vi "Parse INCAR.vi"(8 "error in (no error)":errorcluster, 11 "INCAR File":path=path "C:/Users/Chris B/Documents/Ab Initio/Vasp Calculations/Batch4_20130519/1_Again") -> (0 "error out":errorcluster, 1 "INCAR ID":string, 2 "INCAR Raw Commands":T2(array[cluster]), 3 "INCAR Summary":T1, 5 "Allow Relaxation?":bool)   [LabVIEW 2010]
uses:
  <vilib>/Utility/file.llb/Read From Spreadsheet File (string).vi
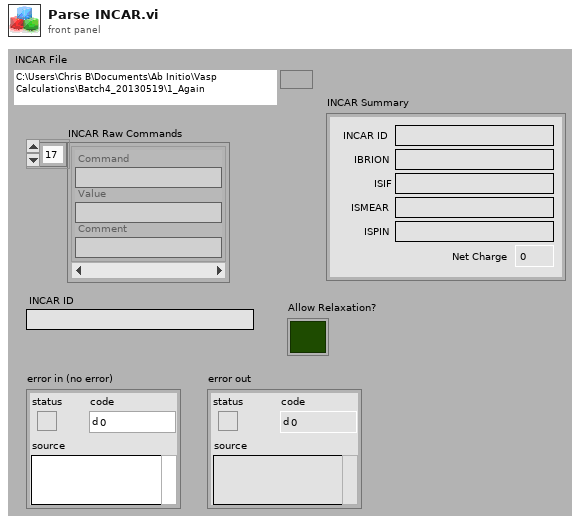
[diagram p1: front panel]
types:
  T1 = cluster{"INCAR ID":string, "IBRION":string, "ISIF":string, "ISMEAR":string, "ISPIN":string, "Net Charge":i32}
  T2 = cluster{"Command":string, "Value":string, "Comment":string}[]
  T3 = cluster{"trimmed string":string, "trimmed string":string, "trimmed string":string}
  T4 = cluster{"trimmed string":string, "trimmed string":string, "trimmed string":string}[]
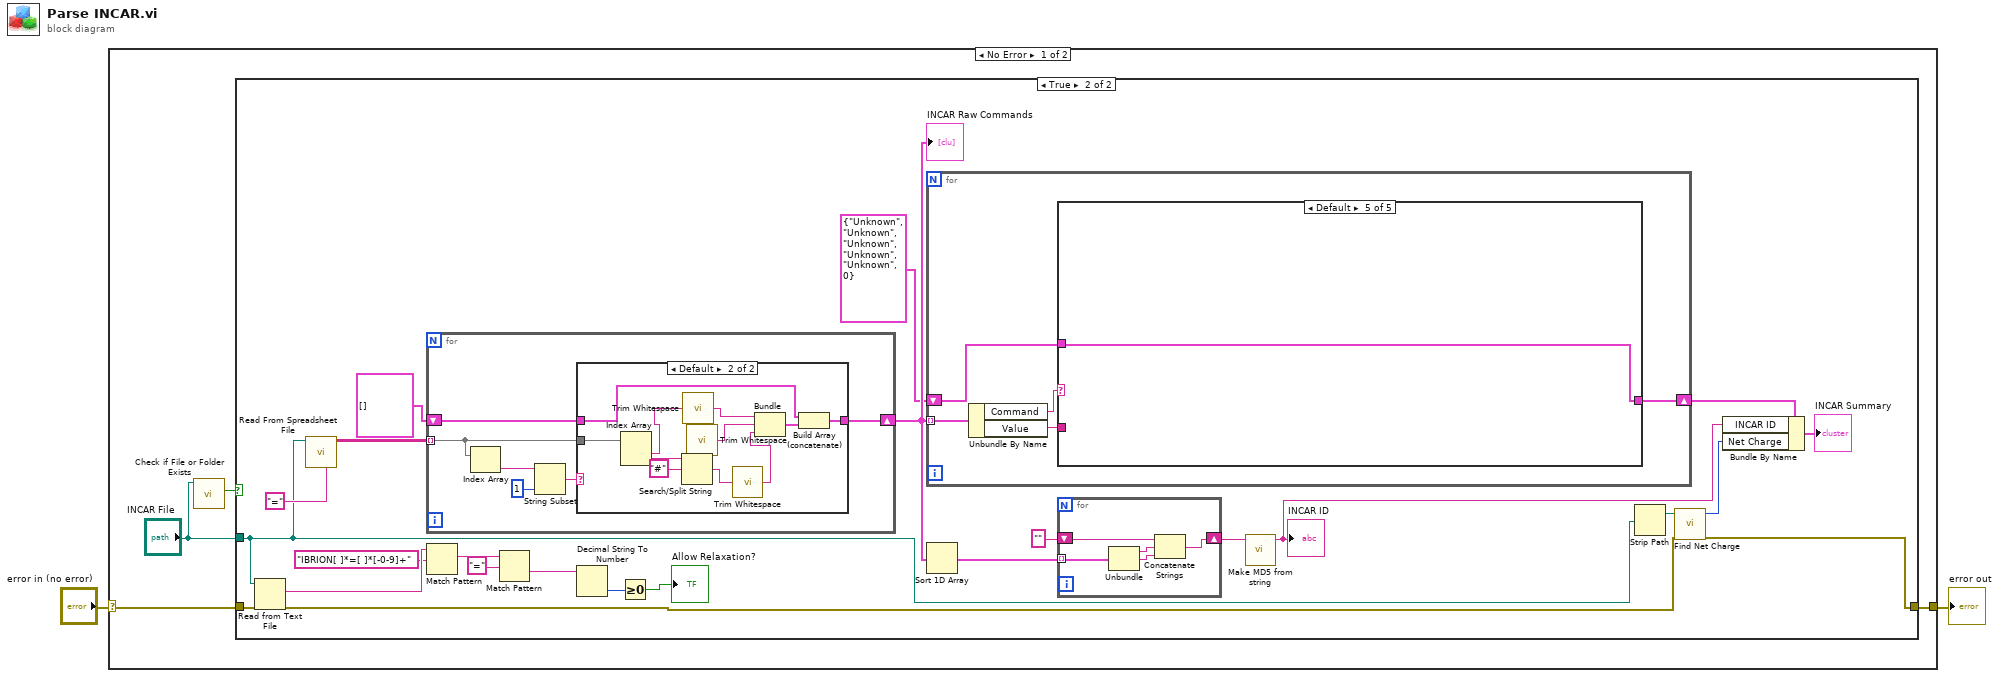
[diagram p0: block diagram]
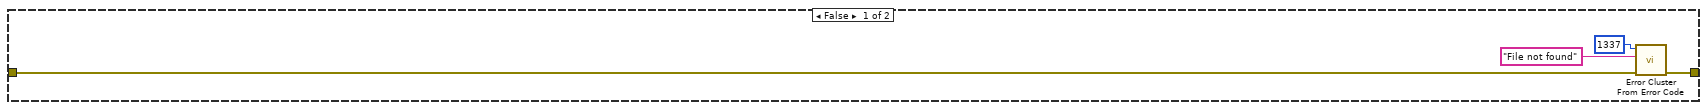
[diagram p2: hidden frame]
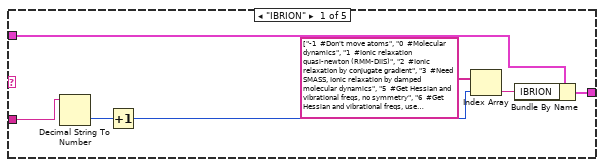
[diagram p3: hidden frame]
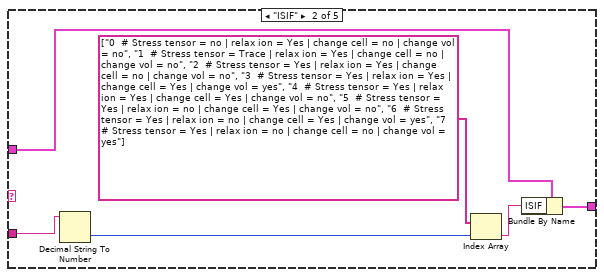
[diagram p4: hidden frame]
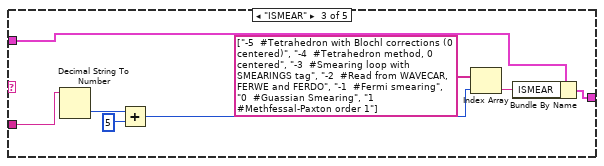
[diagram p5: hidden frame]
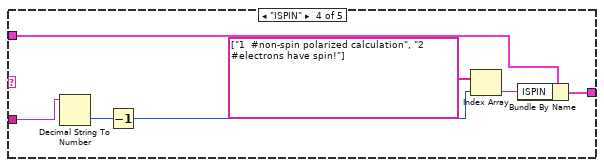
[diagram p6: hidden frame]
diagram:
  n1 = case shown="No Error" "error in (no error)" {
    selector: "error in (no error)" -> [w6 w93]
    tunnel: [w3 w93] -> w1
    frame No Error {
      n2 = call <vilib>:"Check if File or Folder Exists.vi"("path"="INCAR File") -> ("file or folder exists?"=w4:bool)  [unwired: 8 in, 2 out]
      n3 = case shown="True" w4 {
        tunnel: w6 -> [w8 w14]
        tunnel: "INCAR File" -> [_ w13]
        tunnel: [w7 w12] -> w3
        frame False {
          n4 = call <vilib>:"Error Cluster From Error Code.vi"("error in (no error)"=w8, "error message (\"\")"="File not found" ("error message (\"\")"), "error code (0)"=1337) -> ("error out"=w7:errorcluster)  [unwired: 6 in]
        }
        frame True {
          n5 = Read from Text File(file (use dialog)=w13, error in=w14) -> (text=w34:string, error out=w11:errorcluster)  [unwired: 2 in, 2 out]
          n6 = call-poly <vilib>:"Read From Spreadsheet File.vi"("delimiter (\\t)"="=" ("delimiter (\\t)"), "file path (dialog if empty)"=w13) -> ("all rows"=w26:string[][])  [unwired: 5 in, 4 out]
          n7 = for {
            tunnel: w26 -> [w74] mode=indexing
            shift-right: [w76] -> w22
            shift-left: T2 [] ("INCAR Raw Commands 2") -> [w75]
            n8 = Index Array(array=w74) -> (element=w79:string)  [unwired: 1 in]
            n9 = String Subset(string=w79, length (rest)=1 ("length (rest)")) -> (substring=w77:string)  [unwired: 1 in]
            n10 = case shown="Default" w77 {
              tunnel: w74 -> [_ w87]
              tunnel: [w80 w89] -> w76
              tunnel: w75 -> [w80 w88]
              frame "", "#" {
              }
              frame Default {
                n11 = Index Array(array=w87) -> (element #1=w82:string, element #2=w92:string)  [unwired: 2 in]
                n12 = Search/Split String(string=w92, search string/char (-)="#") -> (substring before match=w86:string, match + rest of string=w84:string)  [unwired: 1 in, 1 out]
                n13 = call <vilib>:"Trim Whitespace.vi"("string"=w82) -> ("trimmed string"=w81:string)  [unwired: 1 in]
                n14 = call <vilib>:"Trim Whitespace.vi"("string"=w86) -> ("trimmed string"=w85:string)  [unwired: 1 in]
                n15 = call <vilib>:"Trim Whitespace.vi"("string"=w84) -> ("trimmed string"=w83:string)  [unwired: 1 in]
                n16 = Bundle("trimmed string"=w81, "trimmed string"=w85, "trimmed string"=w83) -> (w90:T3)  [unwired: 1 in]
                n17 = Build Array (concatenate)(w88, w90) -> (w89:T4)
              }
            }
          }
          "INCAR Raw Commands" <- w22
          n18 = Match Pattern(string=w34, regular expression="IBRION[ ]*=[ ]*[-0-9]+") -> (match substring=w32:string)  [unwired: 1 in, 3 out]
          n19 = Match Pattern(string=w32, regular expression="=") -> (after substring=w30:string)  [unwired: 1 in, 3 out]
          n20 = Decimal String To Number(string=w30) -> (number=w29:i32)  [unwired: 2 in, 1 out]
          n21 = Greater Or Equal To 0?(x=w29) -> (x >= 0?=→"Allow Relaxation?":bool)
          n22 = for {
            tunnel: w22 -> [w39] mode=indexing
            shift-right: [w35] -> w19
            shift-left: T1 {"INCAR ID"="Unknown", "IBRION"="Unknown", "ISIF"="Unknown", "ISMEAR"="Unknown", "ISPIN"="Unknown", "Net Charge"=0} ("INCAR Summary 2") -> [w36]
            n23 = Unbundle By Name(w39) -> ("Command"=w38:string, "Value"=w37:string)
            n24 = case shown="Default" w38 {
              tunnel: w37 -> [w46 w52 w60 w67 _]
              tunnel: w36 -> [w42 w49 w55 w66 w68]
              tunnel: [w40 w47 w53 w65 w68] -> w35
              frame "IBRION" {
                n25 = Decimal String To Number(string=w46) -> (number=w44:i32)  [unwired: 2 in, 1 out]
                n26 = Increment(x=w44) -> (x+1=w43:i32)
                n27 = Index Array(array=string[] ["-1  #Don't move atoms", "0  #Molecular dynamics", "1  #Ionic relaxation quasi-newton (RMM-DIIS)", "2  #Ionic relaxation by conjugate gradient", "3  #Need SMASS, Ionic relaxation by damped molecular dynamics", "5  #Get Hessian and vibrational freqs, no symmetry", "6  #Get Hessian and vibrational freqs, use symmetry", "7  #Get Hessian and phonons by perturbation, no symmetry", "8  #Get Hessian and phonons by perturbation, use symmetry", "44  #Improved Dimer Method"], index=w43) -> (element=w41:string)
                n28 = Bundle By Name(cluster=w42, "IBRION"=w41) -> (w40:T1)
              }
              frame "ISIF" {
                n29 = Decimal String To Number(string=w52) -> (number=w50:i32)  [unwired: 2 in, 1 out]
                n30 = Index Array(array=string[] ["0  # Stress tensor = no | relax ion = Yes | change cell = no | change vol = no", "1  # Stress tensor = Trace | relax ion = Yes | change cell = no | change vol = no", "2  # Stress tensor = Yes | relax ion = Yes | change cell = no | change vol = no", "3  # Stress tensor = Yes | relax ion = Yes | change cell = Yes | change vol = yes", "4  # Stress tensor = Yes | relax ion = Yes | change cell = Yes | change vol = no", "5  # Stress tensor = Yes | relax ion = no | change cell = Yes | change vol = no", "6  # Stress tensor = Yes | relax ion = no | change cell = Yes | change vol = yes", "7  # Stress tensor = Yes | relax ion = no | change cell = no | change vol = yes"], index=w50) -> (element=w48:string)
                n31 = Bundle By Name(cluster=w49, "ISIF"=w48) -> (w47:T1)
              }
              frame "ISMEAR" {
                n32 = Decimal String To Number(string=w60) -> (number=w58:i32)  [unwired: 2 in, 1 out]
                n33 = Add(x=w58, y=5) -> (x+y=w57:i32)
                n34 = Index Array(array=string[] ["-5  #Tetrahedron with Blochl corrections (0 centered)", "-4  #Tetrahedron method, 0 centered", "-3  #Smearing loop with SMEARINGS tag", "-2  #Read from WAVECAR, FERWE and FERDO", "-1  #Fermi smearing", "0  #Guassian Smearing", "1  #Methfessal-Paxton order 1"], index=w57) -> (element=w54:string)
                n35 = Bundle By Name(cluster=w55, "ISMEAR"=w54) -> (w53:T1)
              }
              frame "ISPIN" {
                n36 = Decimal String To Number(string=w67) -> (number=w62:i32)  [unwired: 2 in, 1 out]
                n37 = Decrement(x=w62) -> (x-1=w61:i32)
                n38 = Index Array(array=string[] ["1  #non-spin polarized calculation", "2  #electrons have spin!"], index=w61) -> (element=w64:string)
                n39 = Bundle By Name(cluster=w66, "ISPIN"=w64) -> (w65:T1)
              }
              frame Default {
              }
            }
          }
          n40 = Sort 1D Array(array=w22) -> (sorted array=w25:T2)
          n41 = for {
            tunnel: w25 -> [w73] mode=indexing
            shift-right: [w70] -> w23
            shift-left: "" -> [w69]
            n42 = Unbundle(w73) -> ("Command"=w72:string, "Value"=w71:string)  [unwired: 1 out]
            n43 = Concatenate Strings(w69, w72, w71) -> (w70:string)
          }
          n44 = call "Make MD5 from string.vi"("String"=w23) -> ("MD5 message-digest"=w16:string)  [unwired: 10 in]
          "INCAR ID" <- w16
          n45 = Strip Path(path=w13) -> (stripped path=w15:path)  [unwired: 1 out]
          n46 = call "Find Net Charge.vi"("error in (no error)"=w11, "DFT Path"=w15) -> ("error out"=w12:errorcluster, "Net Charge"=w18:i32)  [unwired: 7 in, 1 out]
          n47 = Bundle By Name(cluster=w19, "INCAR ID"=w16, "Net Charge"=w18) -> (→"INCAR Summary":T1)
        }
      }
    }
    frame Error {
    }
  }
  "error out" <- w1
